vi "NI VeriStand - Get Item Children.vi"(8 "error in (no error)":errorcluster, 11 "Item Ref in":T1 format="%.0x") -> (0 "error out":errorcluster, 2 "Child Refs":T1[](array[typedef]) format="%.0x", 3 "Item Ref out":T1 format="%.0x", 4 "Found":bool)   [LabVIEW 2026, in "Custom Devices Storage.lvlib"]
uses:
  Custom Devices Storage.lvlib
  <vilib>/NI VeriStand/Custom Device API/Custom Device Item Ref.ctl
  C:/Users/Administrator/Desktop/Jatin/All DNC DLLs/NationalInstruments.VeriStand.SystemDefinitionAPI.dll
  Jatin/All DNC DLLs/NationalInstruments.VeriStand.SystemDefinitionAPI.dll
  <vilib>/NI VeriStand/Custom Device API/Custom Device API.lvlib
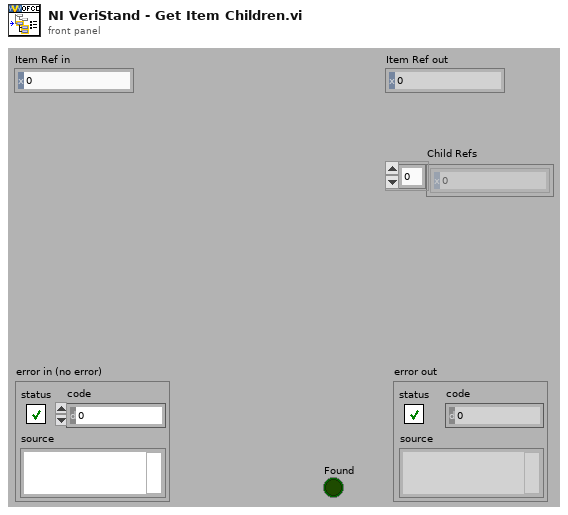
[diagram p1: front panel]
types:
  T1 = typedef "Custom Device API.lvlib/Custom Device Item Ref.ctl" = u64
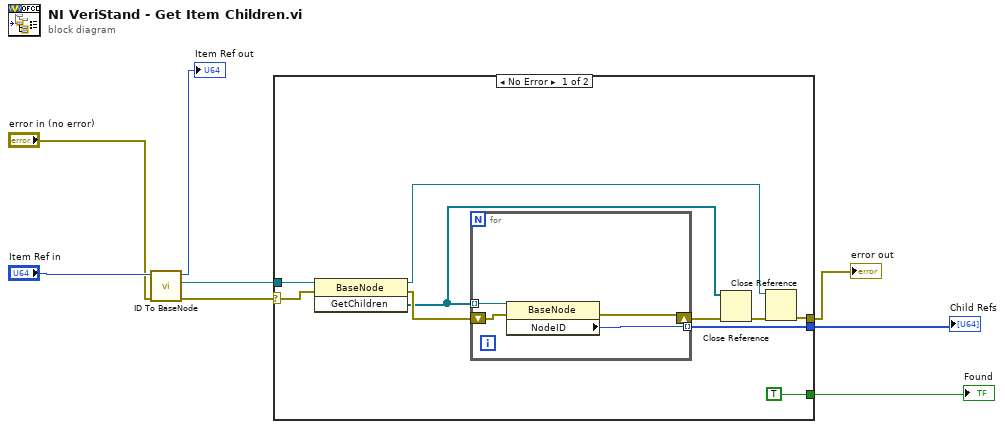
[diagram p0: block diagram]
diagram:
  n1 = call "ID To BaseNode.vi"("error in (no error)"="error in (no error)", "ID in"="Item Ref in") -> ("error out"=w6:errorcluster, "NationalInstruments.VeriStand.SystemDefinitionAPI.BaseNode"=w5:refnum<k39>, "ID out"=→"Item Ref out":u64)  [unwired: 7 in]
  n2 = case shown="No Error" w6 {
    selector: w6 -> [w17 w23]
    tunnel: w5 -> [w18 _]
    tunnel: [w15 _] -> w3
    tunnel: [TRUE _] -> w2
    tunnel: [w10 w23] -> w1
    frame No Error {
      n3 = invoke class="BaseNode" method="GetChildren"(reference=w18, error in=w17) -> (reference out=w9:refnum<k39>, error out=w16:errorcluster, "GetChildren"=w12:refnum<k39>[])  [unwired: 1 in]
      n4 = for {
        shift-right: [w20] -> w13
        shift-left: w16 -> [w21]
        tunnel: w12 -> [w22] mode=indexing
        tunnel: [w19] -> w15 mode=indexing
        n5 = property class="BaseNode"(reference=w22, error in=w21) -> (error out=w20:errorcluster, "NodeID"=w19:u64)  [unwired: 1 out]
      }
      n6 = Close Reference(reference=w12, error in (no error)=w13) -> (error out=w11:errorcluster)
      n7 = Close Reference(reference=w9, error in (no error)=w11) -> (error out=w10:errorcluster)
    }
    frame Error {
    }
  }
  "error out" <- w1
  "Found" <- w2
  "Child Refs" <- w3
